vi "AlliGator Set Phasor Map Color & Cursor Arrays.vi"(8 "Error In":errorcluster, 9 "Array in":refnum<vi>, 11 "Phasor Graph":refnum<vi>) -> (0 "Error Out":errorcluster)   [LabVIEW 2021, in "AlliGator Phasor Plot Color Map.lvlib"]
doc: "Updates color map based on stored vertices and colors."
uses:
  AlliGator Phasor Plot Color Map.lvlib
panel:
  # "see the AlliGator License on the block diagram (Ctrl+E or Window:Show Block Diagram)"
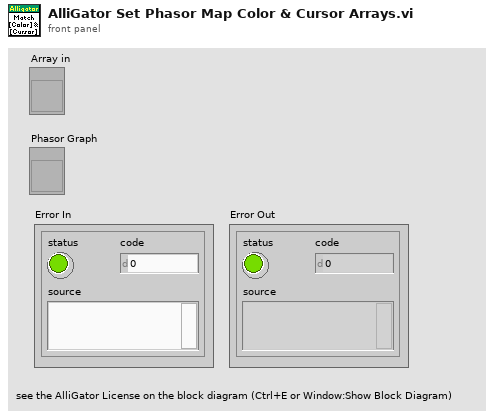
[diagram p1: front panel]
types:
  T1 = cluster{"Name":string, "Color":u32, "Style":u8, "Point Style":u8, "Name Visible":bool, "Allow Drag":bool, "Cursor Mode":u32, "Plot":i32, "Index":i32, "Position":cluster{"X":dbl, "Y":dbl}, "X Scale":u32, "Y Scale":u32, "Watch Plots":i32[], "Watch All Plots":bool, "Plot Area":i32, "Label Offset":cluster{"X":dbl, "Y":dbl}}
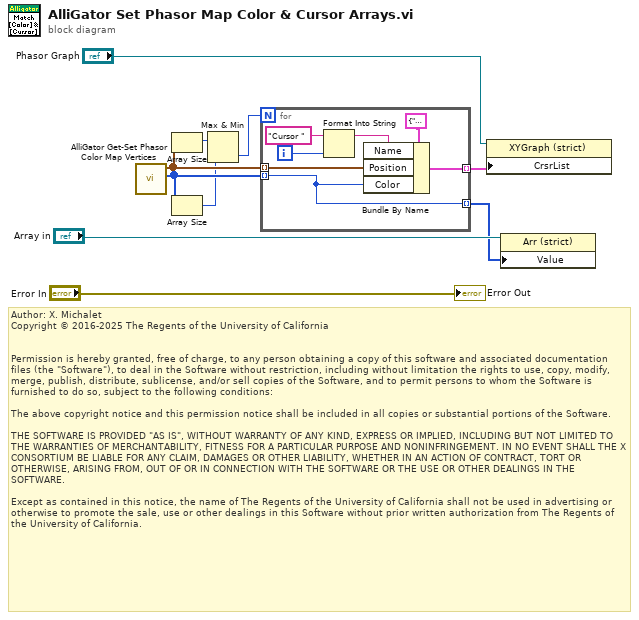
[diagram p0: block diagram]
diagram:
  # "Author: X. Michalet\nCopyright © 2016-2025 The Regents of the University of California\n \n\nPermission is hereby granted, free of charge, to any person obtaining a copy of this software and associated documentation files (the \"Software\"), to deal in the Software without restriction, including without limitation the rights to use, copy, modify, merge, publish, distribute, sublicense, and/or sell copies of the Software, and to permit persons to whom the Software is furnished to do so, subject to the following conditions:\n\nThe above copyright notice and this permission notice shall be included in all copies or substantial portions of the Software.\n\nTHE SOFTWARE IS PROVIDED \"AS IS\", WITHOUT WARRANTY OF ANY KIND, EXPRESS OR IMPLIED, INCLUDING BUT NOT LIMITED TO THE WARRANTIES OF MERCHANTABILITY, FITNESS FOR A PARTICULAR PURPOSE AND NONINFRINGEMENT. IN NO EVENT SHALL THE X CONSORTIUM BE LIABLE FOR ANY CLAIM, DAMAGES OR OTHER LIABILITY, WHETHER IN AN ACTION OF CONTRACT, TORT OR OTHERWISE, ARISING FROM, OUT OF OR IN CONNECTION WITH THE SOFTWARE OR THE USE OR OTHER DEALINGS IN THE SOFTWARE.\n\nExcept as contained in this notice, the name of The Regents of the University of California shall not be used in advertising or otherwise to promote the sale, use or other dealings in this Software without prior written authorization from The Regents of the University of California."
  n1 = call "AlliGator Get-Set Phasor Color Map Vertices.vi"() -> ("Color Array out"=w5:u32[], "Vertices out"=w6:cluster{"X":dbl, "Y":dbl}[])  [unwired: 8 in, 2 out]
  n2 = Array Size(array=w6) -> (size(s)=w4:i32)
  n3 = Array Size(array=w5) -> (size(s)=w3:i32)
  n4 = Max & Min(x=w4, y=w3) -> (min(x,y)=w2:i32)  [unwired: 1 out]
  n5 = for {
    N: w2 -> [_]
    tunnel: w6 -> [w14] mode=indexing
    tunnel: w5 -> [w11] mode=indexing
    tunnel: [w12] -> w8 mode=indexing
    tunnel: [w11] -> w1 mode=indexing
    i -> [w17]
    n6 = Format Into String(initial string="Cursor ", w17) -> (resulting string=w15:string)  [unwired: 2 in, 1 out]
    n7 = Bundle By Name(cluster=T1 {"Name"="", "Color"=0, "Style"=8, "Point Style"=1, "Name Visible"=FALSE, "Allow Drag"=TRUE, "Cursor Mode"=0, "Plot"=0, "Index"=0, "Position"={"X"=0.0, "Y"=0.0}, "X Scale"=0, "Y Scale"=0, "Watch Plots"=[], "Watch All Plots"=FALSE, "Plot Area"=0, "Label Offset"={"X"=0.0, "Y"=0.0}} ("Cluster"), "Name"=w15, "Position"=w14, "Color"=w11) -> (w12:T1)
  }
  n8 = property class="XYGraph (strict)"(reference="Phasor Graph", "CrsrList"=w8) -> ()  [unwired: 1 in, 2 out]
  n9 = property class="Arr (strict)"(reference="Array in", "Value"=w1) -> ()  [unwired: 1 in, 2 out]
  "Error Out" <- "Error In"
